vi "Items Above Range.vi"(9 "map index":i32, 10 "Location Translation":cluster{"dst":i64, "src":i64, "rng":i64}, 11 "Initial Items":cluster{"strt":i64, "rng":i64}) -> (2 "Keep Items?":bool, 3 "Items Above Range":cluster{i64, "lower limit":i64})   [LabVIEW 2023, in "d5.lvlib"]
uses:
  d5.lvlib
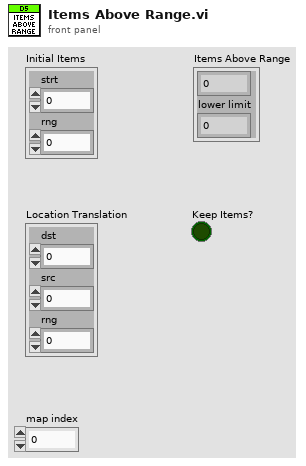
[diagram p1: front panel]
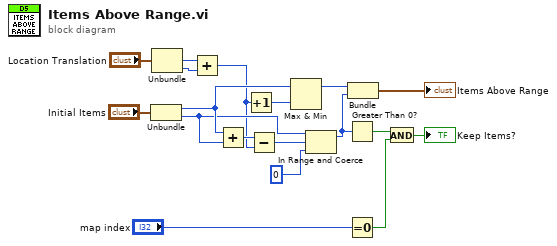
[diagram p0: block diagram]
diagram:
  n1 = Unbundle("Initial Items") -> ("strt"=w5:i64, "rng"=w4:i64)
  n2 = Unbundle("Location Translation") -> ("src"=w17:i64, "rng"=w18:i64)  [unwired: 1 out]
  n3 = Add(x=w17, y=w18) -> (x+y=w3:i64)
  n4 = Add(x=w5, y=w4) -> (x+y=w10:i64)
  n5 = Increment(x=w3) -> (x+1=w14:i64)
  n6 = Subtract(x=w10, y=w3) -> (x-y=w9:i64)
  n7 = Max & Min(x=w5, y=w14) -> (max(x,y)=w6:i64)  [unwired: 1 out]
  n8 = In Range and Coerce(upper limit=w4, x=w9, lower limit=i64 0) -> (coerced(x)=w7:i64)  [unwired: 1 out]
  n9 = Greater Than 0?(x=w7) -> (x > 0?=w13:bool)
  n10 = Equal To 0?(x="map index") -> (x = 0?=w12:bool)
  n11 = Bundle(w6, "rng"=w7) -> (→"Items Above Range":cluster{i64, "rng":i64})  [unwired: 1 in]
  n12 = And(x=w13, y=w12) -> (x .and. y?=→"Keep Items?":bool)
